vi "map_coordinates.vi"(5 "b":dbl, 6 "xi":dbl, 7 "a":dbl, 8 "Error In":errorcluster, 9 "phi_in":dbl, 10 "Xi From":T2, 11 "Parameters":T1) -> (0 "Error Out":errorcluster, 2 "b_pixel":dbl, 3 "a_pixel":dbl)   [LabVIEW 2019]
uses:
  xi_angles_enum_typedef.ctl
  parameters_cluster_typedef.ctl
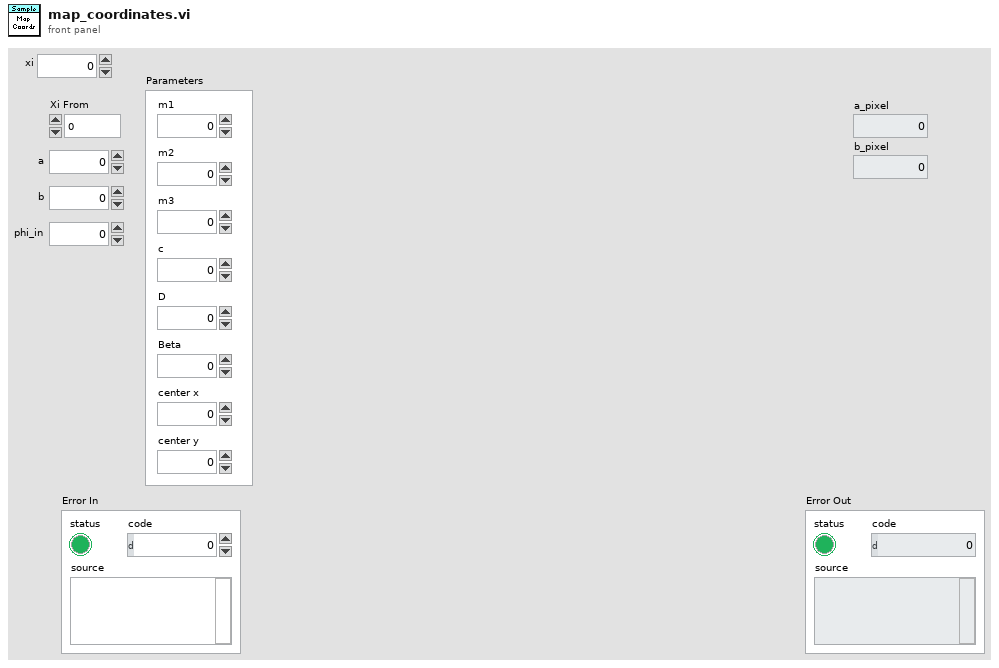
[diagram p1: front panel]
types:
  T1 = typedef "parameters_cluster_typedef.ctl" = cluster{"m1":dbl, "m2":dbl, "m3":dbl, "c":dbl, "D":dbl, "Beta":dbl, "center x":dbl, "center y":dbl}
  T2 = typedef "xi_angles_enum_typedef.ctl" = enum16{"0", "45"}
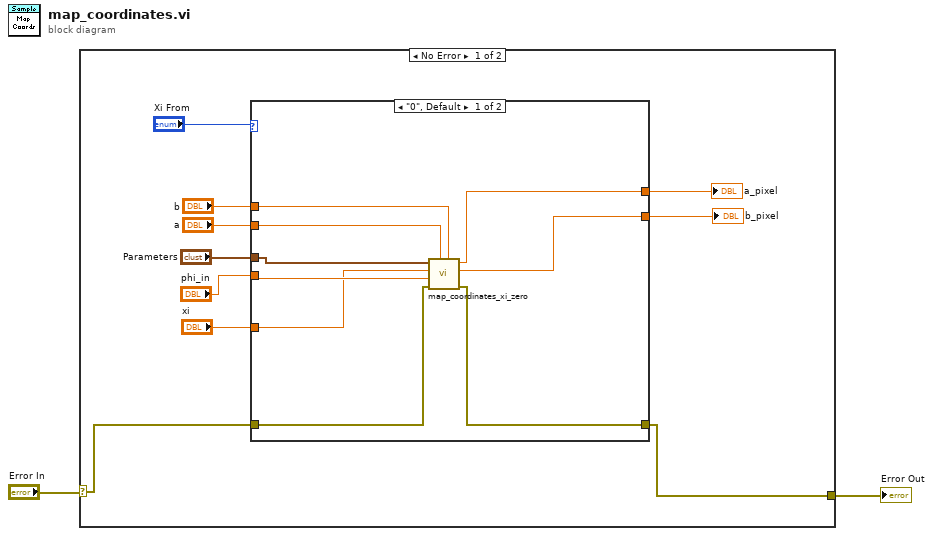
[diagram p0: block diagram]
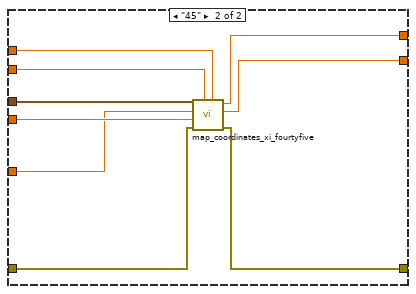
[diagram p2: hidden frame]
diagram:
  n1 = case shown="No Error" "Error In" {
    selector: "Error In" -> [w9 w31]
    tunnel: [w8 w31] -> w1
    frame No Error {
      n2 = case shown="\"0\", Default" "Xi From" {
        tunnel: [w21 w30] -> w11
        tunnel: [w20 w29] -> w10
        tunnel: w9 -> [w15 w28]
        tunnel: [w14 w27] -> w8
        tunnel: "phi_in" -> [w16 w26]
        tunnel: "Parameters" -> [w17 w25]
        tunnel: "b" -> [w19 w24]
        tunnel: "a" -> [w18 w23]
        tunnel: "xi" -> [w13 w22]
        frame "0", Default {
          n3 = call "map_coordinates_xi_zero.vi"("b"=w19, "a"=w18, "Error In"=w15, "phi_in"=w16, "xi"=w13, "Parameters"=w17) -> ("Error Out"=w14:errorcluster, "b_pixel"=w20:dbl, "a_pixel"=w21:dbl)  [unwired: 3 in]
        }
        frame "45" {
          n4 = call "map_coordinates_xi_fourtyfive.vi"("b"=w24, "a"=w23, "Error In"=w28, "phi_in"=w26, "xi"=w22, "Parameters"=w25) -> ("Error Out"=w27:errorcluster, "b_pixel"=w29:dbl, "a_pixel"=w30:dbl)  [unwired: 3 in]
        }
      }
      "a_pixel" <- w11
      "b_pixel" <- w10
    }
    frame Error {
    }
  }
  "Error Out" <- w1
